vi "Open.vi"   [LabVIEW 2011]
uses:
  LMH-PS4.lvlib
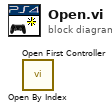
[diagram p0: block diagram]
diagram:
  n1 = call "Open By Index.vi"() -> ()  [unwired: 9 in, 3 out]
  n2 = call "Open First Controller.vi"() -> ()  [unwired: 9 in, 3 out]
